vi "Report Errors.vi"(8 "Error Index":i32, 9 "Channel Index":i32, 10 "stop":bool, 11 "RT Data":T1 {"End System Handle" format="%x"; "Label Transfer Config"."Block Data Refs"."Data Reference" format="%.0x"; "Status Config"."Hardware Out Dur Reference" format="%.0x"; "Status Config"."Hardware In Dur Reference" format="%.0x"; "Status Config"."Hardware Out Count Reference" format="%.0x"; "Status Config"."Hardware In Count Reference" format="%.0x"; "Status Config"."Error Data Reference" format="%.0x"; "Hardware Output Tx Channels"."Message Settings"."Transmit Channel Data Reference" format="%.0x"; "Hardware Output Tx Channels"."Message Settings"."Queue Transmit Channel" format="%.0x"; "Hardware Output Tx Channels"."Message Settings"."Driver Data"."Num Bits" min=1 max=32; "Hardware Output Tx Channels"."Message Settings"."Block Data Refs"."Data Reference" format="%.0x"; "Hardware Output Tx Channels"."Rx Com Udp Port"."Handle" format="%08x"; "Hardware Output Tx Channels"."Tx Com Udp Port"."Handle" format="%08x"; "Hardware Input Rx Channels"."Message Settings"."Transmit Channel Data Reference" format="%.0x"; "Hardware Input Rx Channels"."Message Settings"."Queue Transmit Channel" format="%.0x"; "Hardware Input Rx Channels"."Message Settings"."Driver Data"."Num Bits" min=1 max=32; "Hardware Input Rx Channels"."Message Settings"."Block Data Refs"."Data Reference" format="%.0x"; "Hardware Input Rx Channels"."Rx Com Udp Port"."Handle" format="%08x"; "Hardware Input Rx Channels"."Tx Com Udp Port"."Handle" format="%08x"}) -> ()   [LabVIEW 2013, in "AIT 664 Custom Device.lvlib"]
uses:
  AIT 664 Custom Device.lvlib
  RT Controls/AIT 664  - RT Data.ctl
  RT Controls/AIT 664 - RT Hardware Channel.ctl
  RT Controls/AIT 664 - RT Message Settings.ctl
  <vilib>/NI Veristand/Custom Device API/Block Data Reference.ctl
  <vilib>/NI Veristand/Custom Device API/Data Reference.ctl
  RT Controls/AIT 664 - Driver Data.ctl
  Controls and Global/Start Bit.ctl
  Controls and Global/Number of Bits.ctl
  <vilib>/NI Veristand/Custom Device API/Custom Device Item Ref.ctl
  <userlib>/ARINC 664/AIT 664 Controls/General/Message Port.ctl
  <userlib>/ARINC 664/AIT 664 Controls/General/Direction.ctl
  <userlib>/ARINC 664/AIT 664 Controls/General/Message Port Type.ctl
  System Explorer/Controls/664 - Sampling Type.ctl
  RT Controls/Status Channels Config.ctl
  RT Controls/FIFO.ctl
  RT Controls/Label Transfer Config.ctl
  SubVIs/Error/Print Error.vi
  <vilib>/NI Veristand/Custom Device Tools/Custom Device Utility Library/Custom Device Utility Library.lvlib
  <vilib>/NI Veristand/Custom Device API/Custom Device API.lvlib
  <userlib>/ARINC 664/AIT 664 API.lvlib
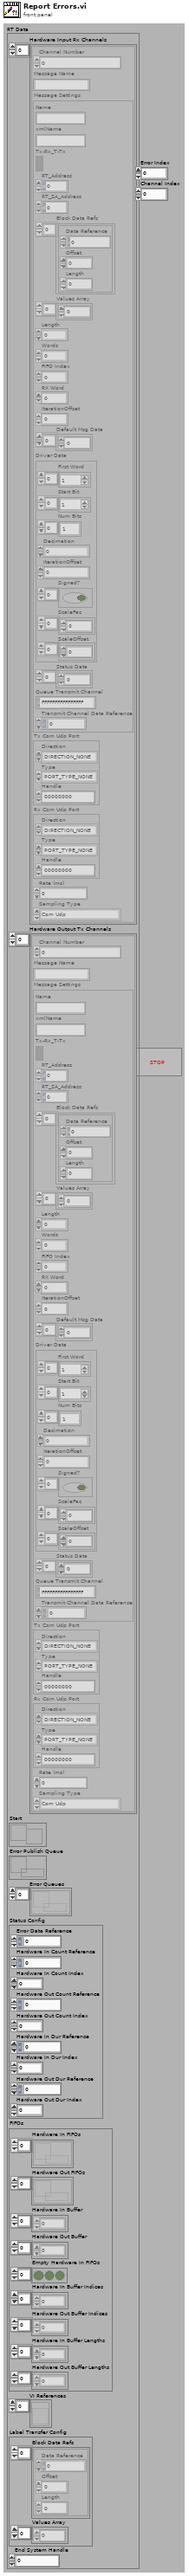
[diagram p1: front panel]
types:
  T1 = typedef "AIT 664 Custom Device.lvlib/AIT 664  - RT Data.ctl" = cluster{"Hardware Input Rx Channels":T2[], "Hardware Output Tx Channels":T2[], "Start":refnum<notifier>, "Error Publish Queue":refnum<queue>, "Error Queues":refnum<queue>[], "Status Config":T14, "FIFOs":T15, "VI References":refnum<vi>[], "Label Transfer Config":T16, "End System Handle ":u64}
  T2 = typedef "AIT 664 Custom Device.lvlib/AIT 664 - RT Hardware Channel.ctl" = cluster{"Channel Number":u16, "Message Name":string, "Message Settings":T3, "Tx Com Udp Port":T10, "Rx Com Udp Port":T10, "Rate (ms)":u32, "Sampling Type":T13}
  T3 = typedef "AIT 664 Custom Device.lvlib/AIT 664 - RT Message Settings.ctl" = cluster{"Name":string, "xmlName":string, "Tx-Rx_T-Tx":bool, "RT_Address":u8, "RT_SA_Address":u8, "Block Data Refs":T4[], "Values Array":dbl[], "Length":i32, "Words":i32, "FIFO Index":i32, "RX Word":u32, "IterationOffset":i32, "Default Msg Data":u8[], "Driver Data":T6, "Status Data":u32[], "Queue Transmit Channel":T9, "Transmit Channel Data Reference":T5}
  T4 = typedef "Custom Device API.lvlib/Block Data Reference.ctl" = cluster{"Data Reference":T5, "Offset":i32, "Length":i32}
  T5 = typedef "Custom Device API.lvlib/Data Reference.ctl" = i32
  T6 = typedef "AIT 664 Custom Device.lvlib/AIT 664 - Driver Data.ctl" = cluster{"First Word":T7[], "Start Bit":T7[], "Num Bits":T8[], "Decimation":i32, "IterationOffset":i32, "Signed?":bool[], "ScaleFac":dbl[], "ScaleOffset":dbl[]}
  T7 = typedef "AIT 664 Custom Device.lvlib/Start Bit.ctl" = i32
  T8 = typedef "AIT 664 Custom Device.lvlib/Number of Bits.ctl" = i32
  T9 = typedef "Custom Device API.lvlib/Custom Device Item Ref.ctl" = u64
  T10 = typedef "AIT 664 API.lvlib/Message Port.ctl" = cluster{"Direction":T11, "Type":T12, "Handle":u64}
  T11 = typedef "AIT 664 API.lvlib/Direction.ctl" = enum16{"DIRECTION_NONE", "DIRECTION_TX", "DIRECTION_RX"}
  T12 = typedef "AIT 664 API.lvlib/Message Port Type.ctl" = enum16{"PORT_TYPE_NONE", "COM_UDP", "SAP_UDP", "SAP_IP", "SAP_MAC", "COTS_MAC", "COTS_MAC_RAW"}
  T13 = typedef "AIT 664 Custom Device.lvlib/664 - Sampling Type.ctl" = enum16{"Com Udp", "Com Udp Queuing", "Sap Udp", "Sap Ip", "Sap Mac", "Unknown"}
  T14 = typedef "AIT 664 Custom Device.lvlib/Status Channels Config.ctl" = cluster{"Error Data Reference":T5, "Hardware In Count Reference":T5, "Hardware In Count Index":i32, "Hardware Out Count Reference":T5, "Hardware Out Count Index":i32, "Hardware In Dur Reference":T5, "Hardware In Dur Index":i32, "Hardware Out Dur Reference":T5, "Hardware Out Dur Index":i32}
  T15 = typedef "AIT 664 Custom Device.lvlib/FIFO.ctl" = cluster{"Hardware In FIFOs":refnum<k33>[], "Hardware Out FIFOs":refnum<k33>[], "Hardware In Buffer":dbl[], "Hardware Out Buffer":dbl[], "Empty Hardware In FIFOs":bool[], "Hardware In Buffer Indices":i32[], "Hardware Out Buffer Indices":i32[], "Hardware In Buffer Lengths":i32[], "Hardware Out Buffer Lengths":i32[]}
  T16 = typedef "AIT 664 Custom Device.lvlib/Label Transfer Config.ctl" = cluster{"Block Data Refs":T4[], "Values Array":dbl[]}
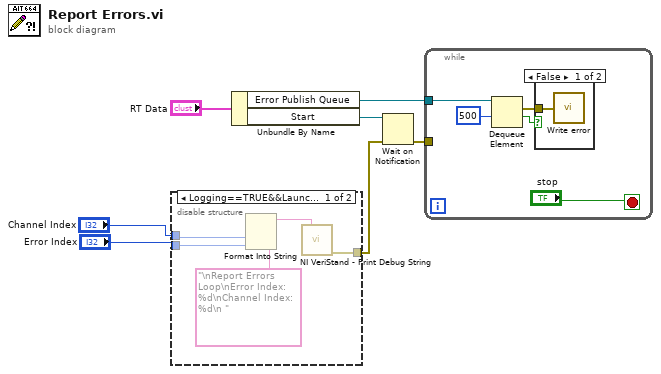
[diagram p0: block diagram]
diagram:
  n1 = disable-structure shown="Logging==TRUE&&LaunchLoopLogging==TRUE" {
    disable-tunnel: "Channel Index" -> [w11 _]
    disable-tunnel: [w9 _] -> w1
    disable-tunnel: "Error Index" -> [w8 _]
    frame condition #0 {
      n2 = Format Into String(format string="\nReport Errors Loop\nError Index: %d\nChannel Index: %d\n ", w11, w8) -> (resulting string=w10:string)  [unwired: 2 in, 1 out]
      n3 = call <vilib>:"NI VeriStand - Print Debug String.vi"("Message"=w10) -> ("error out"=w9:errorcluster)  [unwired: 10 in]
    }
    frame condition #1 (active) {
    }
  }
  n4 = Unbundle By Name("RT Data") -> ("Error Publish Queue"=w5:refnum<queue>, "Start"=w6:refnum<notifier>)
  n5 = Wait on Notification(notifier=w6, error in (no error)=w1) -> (error out=w4:errorcluster)  [unwired: 2 in, 3 out]
  n6 = while {
    tunnel: w4 -> [_]
    tunnel: w5 -> [w17]
    stop <- "stop" stop-if-true
    n7 = Dequeue Element(queue=w17, timeout in ms (-1)=500) -> (element=w16:errorcluster, timed out?=w14:bool)  [unwired: 1 in, 2 out]
    n8 = case shown="False" w14 {
      tunnel: w16 -> [w18 _]
      frame False {
        n9 = call "Write error.vi"("error in (no error)"=w18) -> ()
      }
      frame True {
      }
    }
  }
